vi "Close VI Projects Map References.vi"(8 "Error in":errorcluster caption="Error in (no error)", 11 "VI Projects Map":T1) -> (0 "Error out":errorcluster)   [LabVIEW 2023, in "VIDoc Parsing.lvlib" / "VIDoc Parser.lvclass"]
uses:
  VIDoc Parser.lvclass
  VI Project Map.ctl
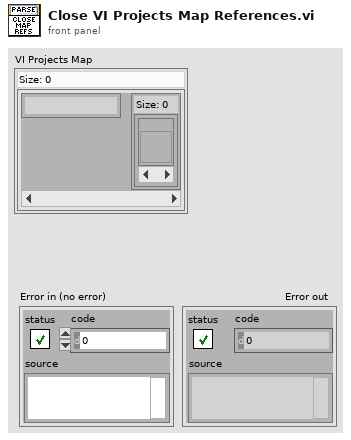
[diagram p1: front panel]
types:
  T1 = typedef "VIDoc Parsing.lvlib/VIDoc Parser.lvclass/VI Project Map.ctl" = map{string, set{refnum<vi>}}
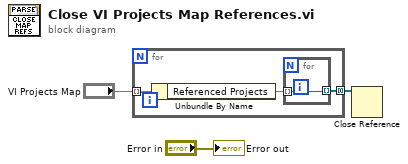
[diagram p0: block diagram]
diagram:
  n1 = for {
    tunnel: "VI Projects Map" -> [w6] mode=indexing
    tunnel: [w4] -> w2 mode=concatenating
    n2 = Unbundle By Name(w6) -> ("Referenced Projects"=w5:set{refnum<vi>})
    n3 = for {
      tunnel: w5 -> [w7] mode=indexing
      tunnel: [w7] -> w4 mode=indexing
    }
  }
  n4 = Close Reference(reference=w2) -> ()  [unwired: 1 in, 1 out]
  "Error out" <- "Error in"
